vi "CTRE_Phoenix_CANdle_SetStandardAnimation.vi"(0 "CTRE_CANdle_DeviceRef":T1, 5 "idx":i32, 7 "speed":dbl, 9 "numLED":i32, 11 "error in":errorcluster, 12 "brightness":dbl, 13 "param4":dbl, 14 "param5":dbl) -> (4 "CTRE_CANdle_DeviceRef":T1, 15 "error out":errorcluster)   [LabVIEW 2020]
uses:
  <vilib>/Rock Robotics/WPI/ThirdParty/Phoenix-LabVIEW/CANdle/Controls/CTRE_Phoenix_CANdle_DeviceRef.ctl
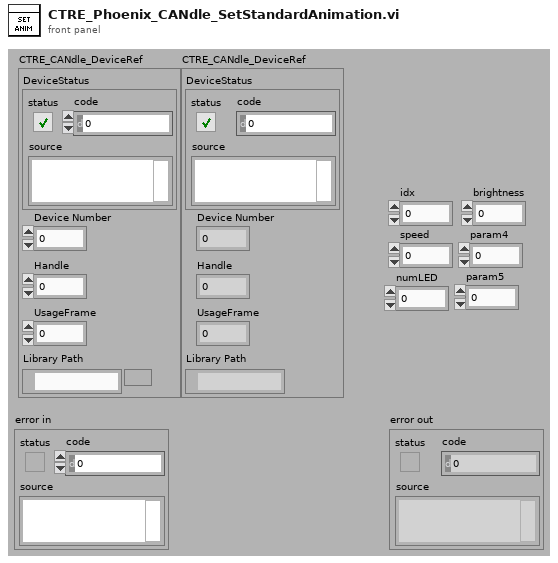
[diagram p1: front panel]
types:
  T1 = typedef "CTRE_Phoenix_CANdle_DeviceRef.ctl" = cluster{"DeviceStatus":errorcluster, "Device Number":u8, "Handle":u64, "UsageFrame":u32, "Library Path":path}
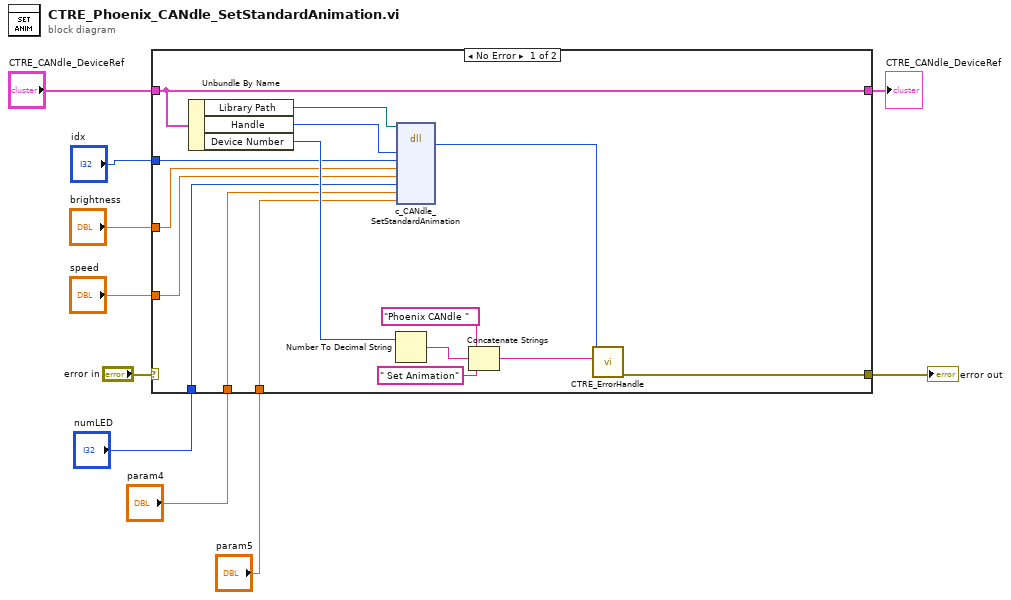
[diagram p0: block diagram]
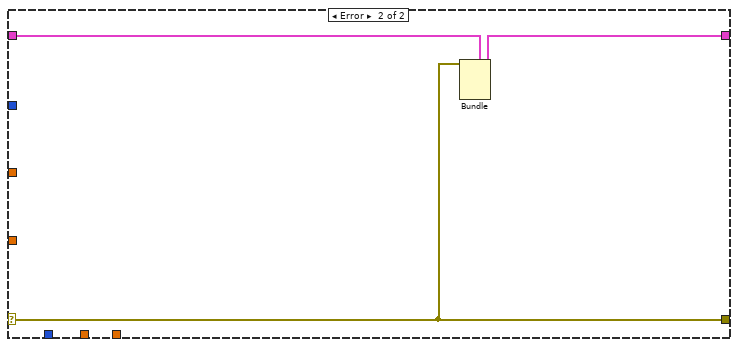
[diagram p2: hidden frame]
diagram:
  n1 = case shown="No Error" "error in" {
    selector: "error in" -> [_ w28]
    tunnel: "CTRE_CANdle_DeviceRef" -> [w20 w29]
    tunnel: [w26 w28] -> w10
    tunnel: [w20 w27] -> w7
    tunnel: "idx" -> [w16 _]
    tunnel: "brightness" -> [w15 _]
    tunnel: "speed" -> [w14 _]
    tunnel: "numLED" -> [w13 _]
    tunnel: "param4" -> [w12 _]
    tunnel: "param5" -> [w11 _]
    frame No Error {
      n2 = Unbundle By Name(w20) -> ("Library Path"=w18:path, "Handle"=w17:u64, "Device Number"=w19:u8)
      n3 = Number To Decimal String(number=w19) -> (decimal integer string=w24:string)  [unwired: 1 in]
      n4 = dll-call lib="?" fn="c_CANdle_SetStandardAnimation"(path in=w18, "handle"=w17, "idx"=w16, "brightness"=w15, "speed"=w14, "numLED"=w13, "param4"=w12, "param5"=w11) -> ("return type"=w22:i32)  [unwired: 9 in, 2 out]
      n5 = Concatenate Strings("Phoenix CANdle " ("string"), w24, " Set Animation" ("string")) -> (w21:string)
      n6 = call <vilib>:"CTRE_ErrorHandle.vi"("origin"=w21, "code"=w22) -> ("error out"=w26:errorcluster)  [unwired: 9 in]
    }
    frame Error {
      n7 = Bundle(cluster=w29, "DeviceStatus"=w28) -> (w27:T1)  [unwired: 4 in]
    }
  }
  "error out" <- w10
  "CTRE_CANdle_DeviceRef" <- w7
